vi "Act Load Data File.vi"(8 "error in (no error)":errorcluster, 10 "File Path":path, 11 "IDE simple in":refnum<class "LF2R IDE.lvclass">) -> (0 "error out":errorcluster, 3 "IDE simple out":refnum<class "LF2R IDE.lvclass">)   [LabVIEW 2018, in "LF2R IDE.lvlib" / "LF2R IDE.lvclass"]
uses:
  LF2R IDE.lvclass
  LF2R IDE.lvclass/LF2R IDE.ctl
  ScintillaNET/ScintillaNET.lvclass
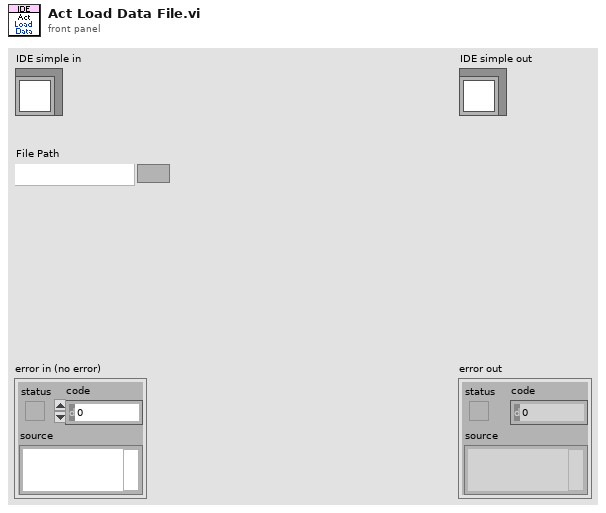
[diagram p1: front panel]
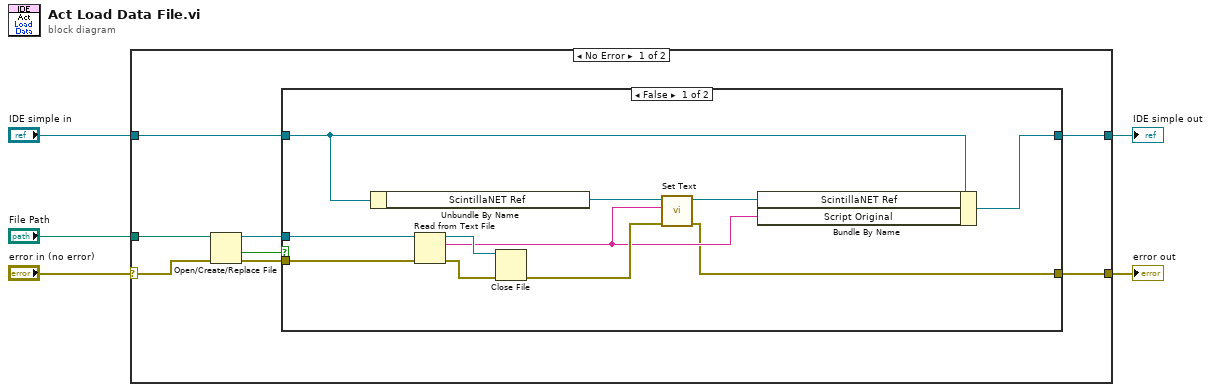
[diagram p0: block diagram]
diagram:
  n1 = case shown="No Error" "error in (no error)" {
    selector: "error in (no error)" -> [w9 w28]
    tunnel: [w7 w28] -> w4
    tunnel: [w8 w27] -> w2
    tunnel: "IDE simple in" -> [w13 w27]
    tunnel: "File Path" -> [w10 _]
    frame No Error {
      n2 = Open/Create/Replace File(file path (use dialog)=w10, error in=w9) -> (refnum out=w12:refnum<file>, cancelled=w6:bool, error out=w11:errorcluster)  [unwired: 4 in]
      n3 = case shown="False" w6 {
        tunnel: w13 -> [w24 w26]
        tunnel: w12 -> [w23 _]
        tunnel: w11 -> [w22 w25]
        tunnel: [w21 w26] -> w8
        tunnel: [w14 w25] -> w7
        frame False {
          n4 = Unbundle By Name(w24) -> ("ScintillaNET Ref"=w18:refnum<class "ScintillaNET.lvclass">)
          n5 = Read from Text File(file (use dialog)=w23, error in=w22) -> (refnum out=w20:refnum<file>, text=w15:string, error out=w19:errorcluster)  [unwired: 2 in, 1 out]
          n6 = Close File(refnum=w20, error in=w19) -> (error out=w17:errorcluster)  [unwired: 1 out]
          n7 = call "Set Text.vi"("error in (no error)"=w17, "Text"=w15, "ScintillaNET in"=w18) -> ("error out"=w14:errorcluster, "ScintillaNET out"=w16:refnum<class "ScintillaNET.lvclass">)  [unwired: 7 in]
          n8 = Bundle By Name(cluster=w24, "ScintillaNET Ref"=w16, "Script Original"=w15) -> (w21:refnum<class "LF2R IDE.lvclass">)
        }
        frame True {
        }
      }
    }
    frame Error {
    }
  }
  "error out" <- w4
  "IDE simple out" <- w2
